vi "check_system_vi.vi"(11 "VIPath":path) -> (2 "x > 0? 2":bool caption="x > 0?", 3 "布尔 2":bool caption="布尔")   [LabVIEW 2020]
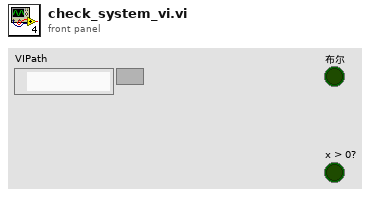
[diagram p1: front panel]
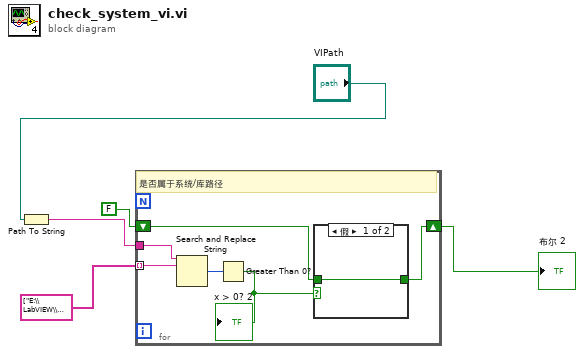
[diagram p0: block diagram]
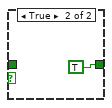
[diagram p2: hidden frame]
diagram:
  n1 = Path To String(path="VIPath") -> (string=w2:string)
  n2 = for {
    tunnel: string[] ["E:\\LabVIEW\\32-bit\\LabVIEW 2020"] ("排除路径输入") -> [w11] mode=indexing
    tunnel: w2 -> [w10]
    shift-right: [w6] -> w1
    shift-left: FALSE -> [w7]
    # "是否属于系统/库路径"
    n3 = Search and Replace String(input string=w10, search string=w11) -> (number of replacements=w9:i32)  [unwired: 6 in, 3 out]
    n4 = Greater Than 0?(x=w9) -> (x > 0?=w8:bool)
    "x > 0? 2" <- w8
    n5 = case shown="假" w8 {
      tunnel: [w12 TRUE] -> w6
      tunnel: w7 -> [w12 _]
      frame False {
      }
      frame True {
      }
    }
  }
  "布尔 2" <- w1
